vi "Periodic Tasks.vi"(8 "error in (no error)":errorcluster) -> ()   [LabVIEW 2023]
doc: "This VI runs in parallel to other tasks. It can contain as many user-defined periodic loops as you need. These can carry out PID or other sorts of timed response."
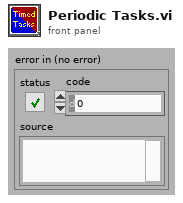
[diagram p1: front panel]
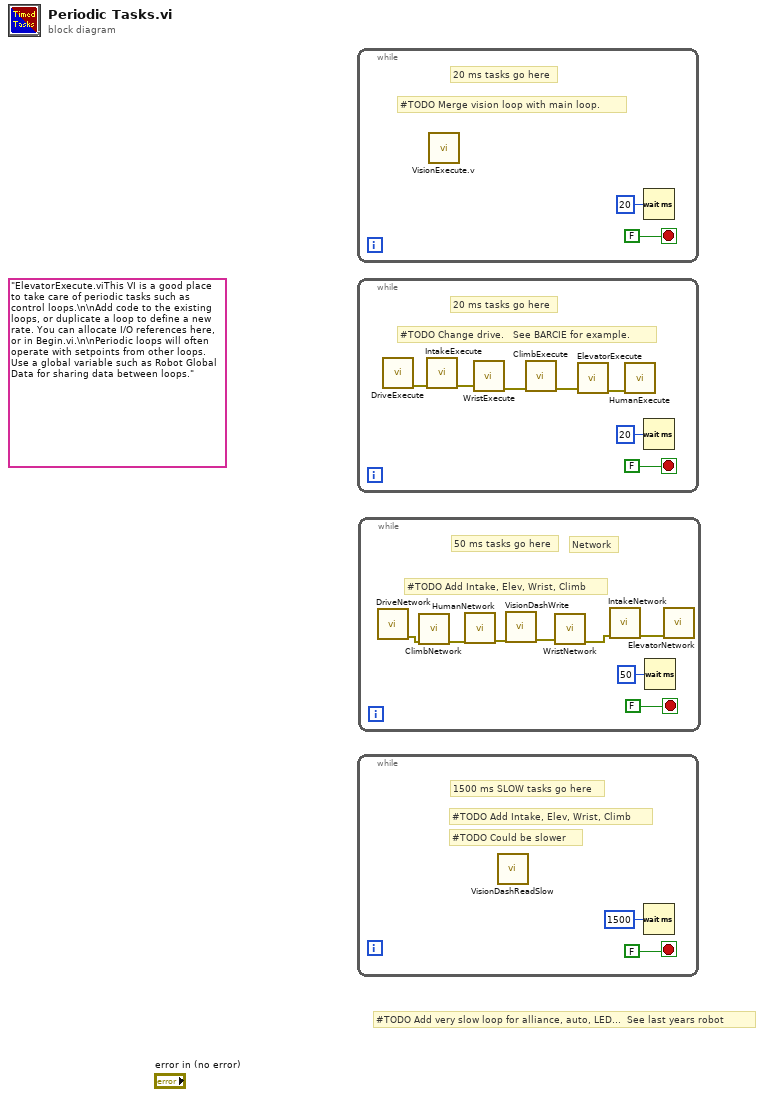
[diagram p0: block diagram]
diagram:
  (unwired) "ElevatorExecute.viThis VI is a good place to take care of periodic tasks such as control loops.\n\nAdd code to the existing loops, or duplicate a loop to define a new rate. You can allocate I/O references here, or in Begin.vi.\n\nPeriodic loops will often operate with setpoints from other loops. Use a global variable such as Robot Global Data for sharing data between loops."
  # "#TODO Add very slow loop for alliance, auto, LED...  See last years robot"
  n1 = while {
    stop <- FALSE stop-if-true
    # "#TODO Merge vision loop with main loop."
    # "20 ms tasks go here"
    n2 = call "VisionExecute.v.vi"() -> ()  [unwired: 11 in, 1 out]
    n3 = Wait (ms)(milliseconds to wait=u32 20) -> ()  [unwired: 1 out]
  }
  n4 = while {
    stop <- FALSE stop-if-true
    # "#TODO Change drive.   See BARCIE for example."
    # "20 ms tasks go here"
    n5 = call "DriveExecute.vi"() -> ("error out"=w7:errorcluster)  [unwired: 11 in]
    n6 = call "IntakeExecute.vi"("error in (no error)"=w7) -> ("error out"=w6:errorcluster)  [unwired: 10 in]
    n7 = call "WristExecute.vi"("error in (no error)"=w6) -> ("error out"=w5:errorcluster)  [unwired: 10 in]
    n8 = call "ClimbExecute.vi"("error in (no error)"=w5) -> ("error out"=w4:errorcluster)  [unwired: 10 in]
    n9 = call "ElevatorExecute.vi"("error in (no error)"=w4) -> ("error out"=w3:errorcluster)  [unwired: 10 in]
    n10 = call "HumanExecute.vi"("error in (no error)"=w3) -> ()  [unwired: 10 in, 1 out]
    n11 = Wait (ms)(milliseconds to wait=u32 20) -> ()  [unwired: 1 out]
  }
  n12 = while {
    stop <- FALSE stop-if-true
    # "#TODO Could be slower"
    # "#TODO Add Intake, Elev, Wrist, Climb"
    # "1500 ms SLOW tasks go here"
    n13 = call "VisionDashReadSlow.vi"() -> ()  [unwired: 11 in, 1 out]
    n14 = Wait (ms)(milliseconds to wait=u32 1500) -> ()  [unwired: 1 out]
  }
  n15 = while {
    stop <- FALSE stop-if-true
    # "#TODO Add Intake, Elev, Wrist, Climb"
    # "Network"
    # "50 ms tasks go here"
    n16 = call "DriveNetwork.vi"() -> ("error out"=w16:errorcluster)  [unwired: 11 in]
    n17 = call "ClimbNetwork.vi"("error in (no error)"=w16) -> ("error out"=w15:errorcluster)  [unwired: 10 in]
    n18 = call "HumanNetwork.vi"("error in (no error)"=w15) -> ("error out"=w17:errorcluster)  [unwired: 10 in]
    n19 = call "VisionDashWrite.vi"("error in (no error)"=w17) -> ("error out"=w14:errorcluster)  [unwired: 10 in]
    n20 = call "WristNetwork.vi"("error in (no error)"=w14) -> ("error out"=w13:errorcluster)  [unwired: 10 in]
    n21 = call "IntakeNetwork.vi"("error in (no error)"=w13) -> ("error out"=w12:errorcluster)  [unwired: 10 in]
    n22 = Wait (ms)(milliseconds to wait=u32 50) -> ()  [unwired: 1 out]
    n23 = call "ElevatorNetwork.vi"("error in (no error)"=w12) -> ()  [unwired: 10 in, 1 out]
  }
